vi "Read SA Pin.vi"(8 "error in (no error)":errorcluster, 11 "CDMA2K_CHP in":refnum<class "CDMA2K_CHP.lvclass">=refnum) -> (0 "error out":errorcluster, 2 "SA Pin":string, 3 "CDMA2K_CHP out":refnum<class "CDMA2K_CHP.lvclass">)   [LabVIEW 2016, in "SeqAuto Evaluations.lvlib" / "CDMA2K_CHP.lvclass"]
uses:
  CDMA2K_CHP.lvclass
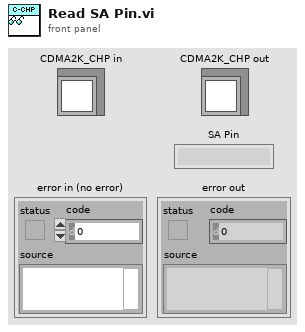
[diagram p1: front panel]
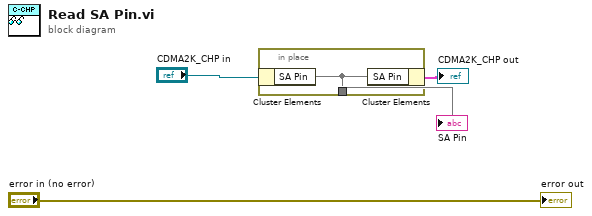
[diagram p0: block diagram]
diagram:
  n1 = in-place {
    in-place-border: [w5] -> w1
    n2 = in-place-cluster #1("CDMA2K_CHP in") -> ("SA Pin"=w5)
    n3 = in-place-cluster #1("SA Pin"=w5) -> (→"CDMA2K_CHP out":cluster{})
  }
  "SA Pin" <- w1
  "error out" <- "error in (no error)"
